vi "PID.vi"(0 "setpoint":dbl format="%.2f", 1 "process variable":dbl format="%.2f", 2 "setpoint high":dbl=100.0 format="%.2f", 3 "setpoint low":dbl format="%.2f", 4 "proportional gain (Kc)":dbl=1.0 format="%.3f", 5 "integral time (Ti, min)":dbl=0.01 format="%.3f", 6 "derivative time (Td, min)":dbl format="%.3f", 7 "dt (s)":dbl=-1.0 format="%.3f", 8 "output high":dbl=100.0 format="%.2f", 9 "reinitialize? (F)":bool, 10 "output low":dbl=-100.0 format="%.2f", 11 "beta":dbl=1.0 format="%.2f", 12 "auto? (T)":bool=TRUE, 13 "linearity":dbl=1.0 format="%.2f", 14 "manual control":dbl format="%.2f", 15 "error in":errorcluster) -> (20 "output":dbl format="%.2f", 26 "error out":errorcluster, 27 "dt out (s)":dbl format="%.3f")   [LabVIEW 2020, in "NI_FunctionBlock Libraries.lvlib"]
doc: "PID algorithm with advanced optional features. This PID algorithm includes the features of the PID VI and also manual mode control with bumpless manual to automatic transitions, non-linear integral action, two degree of freedom control, and error-squared control. You can use this polymorphic VI to operate on a single input value or on an array of input values. The DBL instance can be used to implement a single control loop, whereas the DBL Array instance can be used to implement parallel multi-loop control."
uses:
  <vilib>/functionblocks/NI_FunctionBlock Libraries.lvlib
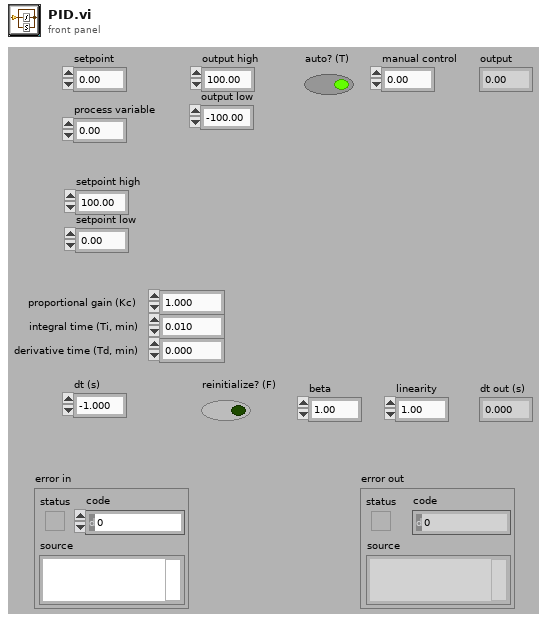
[diagram p1: front panel]
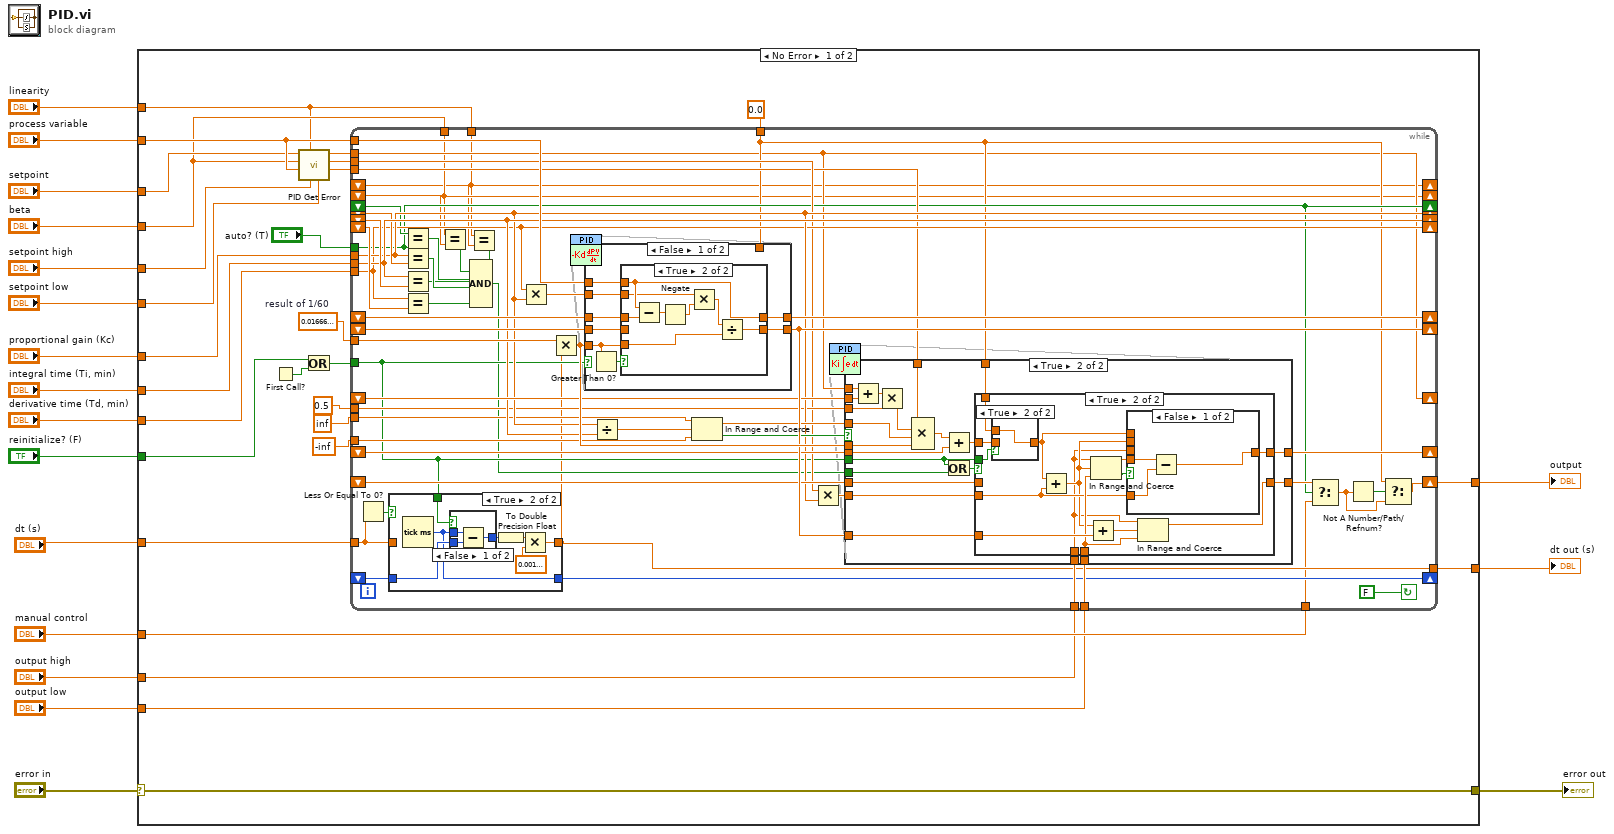
[diagram p0: block diagram]
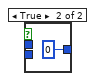
[diagram p3: hidden frame]
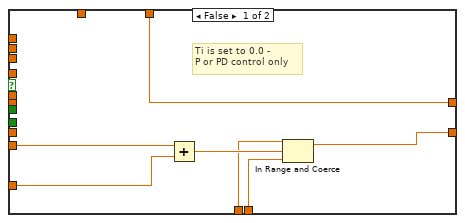
[diagram p4: hidden frame]
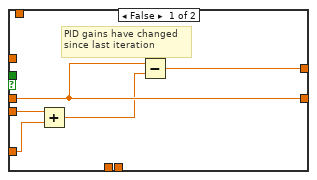
[diagram p5: hidden frame]
diagram:
  n1 = case shown="No Error" "error in" {
    selector: "error in" -> [w19 w190]
    tunnel: "reinitialize? (F)" -> [w46 _]
    tunnel: "dt (s)" -> [w43 _]
    tunnel: [w36 _] -> w16
    tunnel: "manual control" -> [w35 _]
    tunnel: [w34 _] -> w14
    tunnel: "process variable" -> [w33 _]
    tunnel: "setpoint" -> [w32 _]
    tunnel: "beta" -> [w28 _]
    tunnel: "linearity" -> [w27 _]
    tunnel: "output high" -> [w26 _]
    tunnel: "output low" -> [w25 _]
    tunnel: "setpoint high" -> [w24 _]
    tunnel: "setpoint low" -> [w23 _]
    tunnel: "proportional gain (Kc)" -> [w22 _]
    tunnel: "integral time (Ti, min)" -> [w21 _]
    tunnel: "derivative time (Td, min)" -> [w20 _]
    tunnel: [w19 w190] -> w1
    frame No Error {
      w38 = 0.016666666666666666  # result of 1/60
      n2 = First Call?() -> (First Call?: T/F=w45:bool)
      n3 = call <vilib>:"PID Get Error.vi"("setpoint low"=w23, "setpoint high"=w24, "linearity"=w27, "process variable"=w33, "beta"=w28, "setpoint"=w32) -> ("non-linear integral action"=w31:dbl, "error with beta"=w30:dbl, "error"=w29:dbl)  [unwired: 3 in]
      n4 = Or(x=w46, y=w45) -> (x .or. y?=w42:bool)
      n5 = while {
        tunnel: w42 -> [w66]
        shift-left: _ -> [w69]
        shift-right: [w70] -> _
        shift-right: [w77] -> _
        shift-left: _ -> [w78]
        shift-right: [w79] -> _
        shift-left: _ -> [w100]
        shift-right: [w72] -> _
        shift-left: _ -> [w101]
        tunnel: w22 -> [w77]
        tunnel: w21 -> [w79]
        tunnel: w20 -> [w72]
        tunnel: w43 -> [w68]
        tunnel: w26 -> [w96]
        tunnel: w25 -> [w95]
        tunnel: w33 -> [w94]
        shift-right: [w93] -> _
        shift-left: _ -> [w92]
        shift-right: [w91] -> _
        shift-left: _ -> [w84]
        shift-right: [w55] -> w34
        shift-left: _ -> [w90]
        shift-right: [w53] -> _
        shift-left: _ -> [w89]
        shift-right: [w88] -> _
        shift-left: _ -> [w87]
        tunnel: w38 -> [w81]
        tunnel: 0.5 ("y") -> [w76]
        tunnel: inf ("upper limit") -> [w74]
        tunnel: -inf ("lower limit") -> [w75]
        tunnel: w30 -> [w71]
        tunnel: 0.0 -> [w54]
        tunnel: w31 -> [w65]
        shift-right: [w57] -> _
        shift-left: _ -> [w64]
        tunnel: "auto? (T)" -> [w57]
        tunnel: [w61] -> w36
        tunnel: w35 -> [w56]
        tunnel: w29 -> [w53]
        shift-right: [w52] -> _
        shift-left: _ -> [w51]
        tunnel: w28 -> [w52]
        shift-right: [w49] -> _
        shift-left: _ -> [w47]
        tunnel: w27 -> [w49]
        stop <- FALSE continue-if-true
        n6 = Less Or Equal To 0?(x=w68) -> (x <= 0?=w67:bool)
        n7 = case shown="True" w67 {
          tunnel: [w104 w108] -> w61
          tunnel: w69 -> [w103 w107]
          tunnel: [w103 w106] -> w70
          tunnel: w68 -> [w104 _]
          tunnel: w66 -> [_ w105]
          frame False {
          }
          frame True {
            n8 = Tick Count (ms)() -> (millisecond timer value=w106:u32)
            n9 = case shown="False" w105 {
              tunnel: [w114 u32 0] -> w110
              tunnel: w107 -> [w113 _]
              tunnel: w106 -> [w112 _]
              frame False {
                n10 = Subtract(x=w112, y=w113) -> (x-y=w114:u32)
              }
              frame True {
              }
            }
            n11 = To Double Precision Float(number=w110) -> (double precision float=w109:dbl)
            n12 = Multiply(x=w109, y=0.0010000000474974513) -> (x*y=w108:dbl)
          }
        }
        n13 = Equal?(x=w64, y=w57) -> (x = y?=w62:bool)
        n14 = Equal?(x=w77, y=w78) -> (x = y?=w98:bool)
        n15 = Equal?(x=w79, y=w100) -> (x = y?=w97:bool)
        n16 = Equal?(x=w72, y=w101) -> (x = y?=w99:bool)
        n17 = Equal?(x=w52, y=w51) -> (x = y?=w50:bool)
        n18 = Equal?(x=w49, y=w47) -> (x = y?=w48:bool)
        n19 = Compound Arithmetic op=AND(w48, w50, w62, w98, w97, w99) -> (w63:bool)
        n20 = Multiply(x=w72, y=w77) -> (x*y=w83:dbl)
        n21 = Multiply(x=w81, y=w61) -> (x*y=w102:dbl)
        n22 = case shown="False" w66 {
          tunnel: w92 -> [w177 _]
          tunnel: w83 -> [w174 _]
          tunnel: w94 -> [w176 w189]
          tunnel: [w173 w189] -> w93
          tunnel: [w175 w188] -> w91
          tunnel: w84 -> [w171 _]
          tunnel: w102 -> [w170 _]
          tunnel: w54 -> [_ w188]
          frame False {
            n23 = Greater Than 0?(x=w170) -> (x > 0?=w172:bool)
            n24 = case shown="True" w172 {
              tunnel: w177 -> [w179 w185]
              tunnel: w170 -> [_ w184]
              tunnel: w176 -> [_ w182]
              tunnel: [w178 w183] -> w175
              tunnel: w174 -> [_ w180]
              tunnel: [w179 w182] -> w173
              tunnel: w171 -> [w178 _]
              frame False {
                # "dt = 0 min"
              }
              frame True {
                n25 = Subtract(x=w182, y=w185) -> (x-y=w187:dbl)
                n26 = Negate(x=w187) -> (-x=w181:dbl)
                n27 = Multiply(x=w180, y=w181) -> (x*y=w186:dbl)
                n28 = Divide(x=w186, y=w184) -> (x/y=w183:dbl)
              }
            }
          }
          frame True {
          }
        }
        n29 = Divide(x=w77, y=w79) -> (x/y=w82:dbl)
        n30 = In Range and Coerce(upper limit=w74, x=w82, lower limit=w75) -> (coerced(x)=w86:dbl, In Range?=w85:bool)
        n31 = Multiply(x=w71, y=w77) -> (x*y=w80:dbl)
        n32 = case shown="True" w85 {
          tunnel: w53 -> [_ w143]
          tunnel: w89 -> [_ w144]
          tunnel: w87 -> [_ w139]
          tunnel: [w116 w134] -> w88
          tunnel: w86 -> [_ w132]
          tunnel: w80 -> [w121 w137]
          tunnel: [w122 w133] -> w58
          tunnel: w90 -> [_ w135]
          tunnel: w91 -> [w120 w131]
          tunnel: w66 -> [_ w130]
          tunnel: w63 -> [_ w129]
          tunnel: w102 -> [_ w128]
          tunnel: w96 -> [w118 w126]
          tunnel: w95 -> [w117 w127]
          tunnel: w76 -> [_ w125]
          tunnel: w54 -> [w116 w124]
          tunnel: w65 -> [_ w123]
          frame False {
            # "Ti is set to 0.0 -\nP or PD control only"
            n33 = Add(x=w121, y=w120) -> (x+y=w119:dbl)
            n34 = In Range and Coerce(upper limit=w118, x=w119, lower limit=w117) -> (coerced(x)=w122:dbl)  [unwired: 1 out]
          }
          frame True {
            n35 = Add(x=w143, y=w144) -> (x+y=w142:dbl)
            n36 = Multiply(x=w142, y=w125) -> (x*y=w141:dbl)
            n37 = Compound Arithmetic op=MULTIPLY(w123, w141, w132, w128) -> (w140:dbl)
            n38 = Add(x=w140, y=w139) -> (x+y=w138:dbl)
            n39 = Or(x=w130, y=w129) -> (x .or. y?=w136:bool)
            n40 = case shown="True" w136 {
              tunnel: w138 -> [_ w157]
              tunnel: w137 -> [w147 w153]
              tunnel: w135 -> [w149 _]
              tunnel: w130 -> [_ w159]
              tunnel: [w148 w155] -> w134
              tunnel: [w149 w162] -> w133
              tunnel: w131 -> [w146 w161]
              tunnel: w127 -> [_ w160]
              tunnel: w126 -> [_ w151]
              tunnel: w124 -> [_ w158]
              frame False {
                # "PID gains have changed\nsince last iteration"
                n41 = Add(x=w147, y=w146) -> (x+y=w145:dbl)
                n42 = Subtract(x=w149, y=w145) -> (x-y=w148:dbl)
              }
              frame True {
                n43 = case shown="True" w159 {
                  tunnel: w158 -> [_ w169]
                  tunnel: [w168 w169] -> w156
                  tunnel: w157 -> [w168 _]
                  frame False {
                  }
                  frame True {
                  }
                }
                n44 = Add(x=w156, y=w153) -> (x+y=w152:dbl)
                n45 = Add(x=w152, y=w161) -> (x+y=w163:dbl)
                n46 = In Range and Coerce(upper limit=w151, x=w152, lower limit=w160) -> (coerced(x)=w150:dbl, In Range?=w154:bool)
                n47 = case shown="False" w154 {
                  tunnel: w156 -> [_ w167]
                  tunnel: [w164 w167] -> w155
                  tunnel: w150 -> [w166 _]
                  tunnel: w153 -> [w165 _]
                  tunnel: w151 -> [_ _]
                  tunnel: w152 -> [_ _]
                  frame False {
                    n48 = Subtract(x=w166, y=w165) -> (x-y=w164:dbl)
                  }
                  frame True {
                  }
                }
                n49 = In Range and Coerce(upper limit=w151, x=w163, lower limit=w160) -> (coerced(x)=w162:dbl)  [unwired: 1 out]
              }
            }
          }
        }
        n50 = Select(t=w58, s=w57, f=w56) -> (s? t:f=w60:dbl)
        n51 = Not A Number/Path/Refnum?(number/path/refnum=w60) -> (NaN/Path/Refnum?=w59:bool)
        n52 = Select(t=w54, s=w59, f=w60) -> (s? t:f=w55:dbl)
      }
    }
    frame Error {
    }
  }
  "dt out (s)" <- w16
  "output" <- w14
  "error out" <- w1
